vi "PQMain.vi"() -> ()   [LabVIEW 2009]
uses:
  PriorityQueue/Priority.ctl
  PriorityQueue/PriorityQueue.lvclass
  LinkedList/LinkedList.lvclass
panel:
  in  "Demo":enum32{"Basic", "Performance"}(tab)
  out "Message":string
  in  "Next Message":bool
  in  "Exit":bool
  out "data":i32(graph)
  out "generate (ms)":u32
  out "time enque":u32
  out "size":i32
  out "time deque":u32
  out "consume (ms)":u32
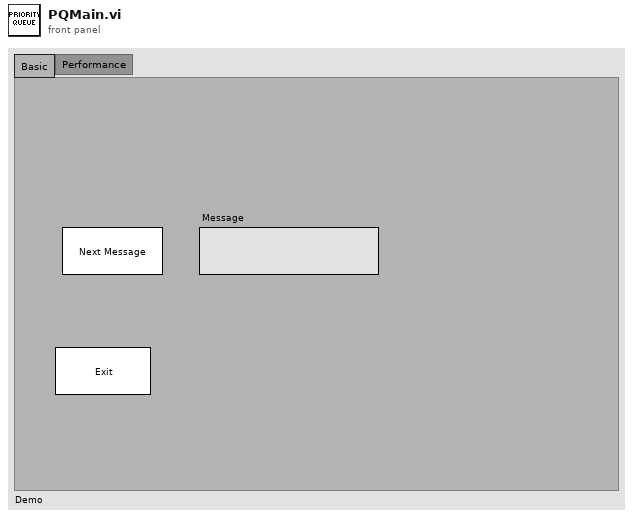
[diagram p1: front panel]
types:
  T1 = typedef "PriorityQueue.lvclass/Priority.ctl" = enum16{"High", "Medium", "Low"}
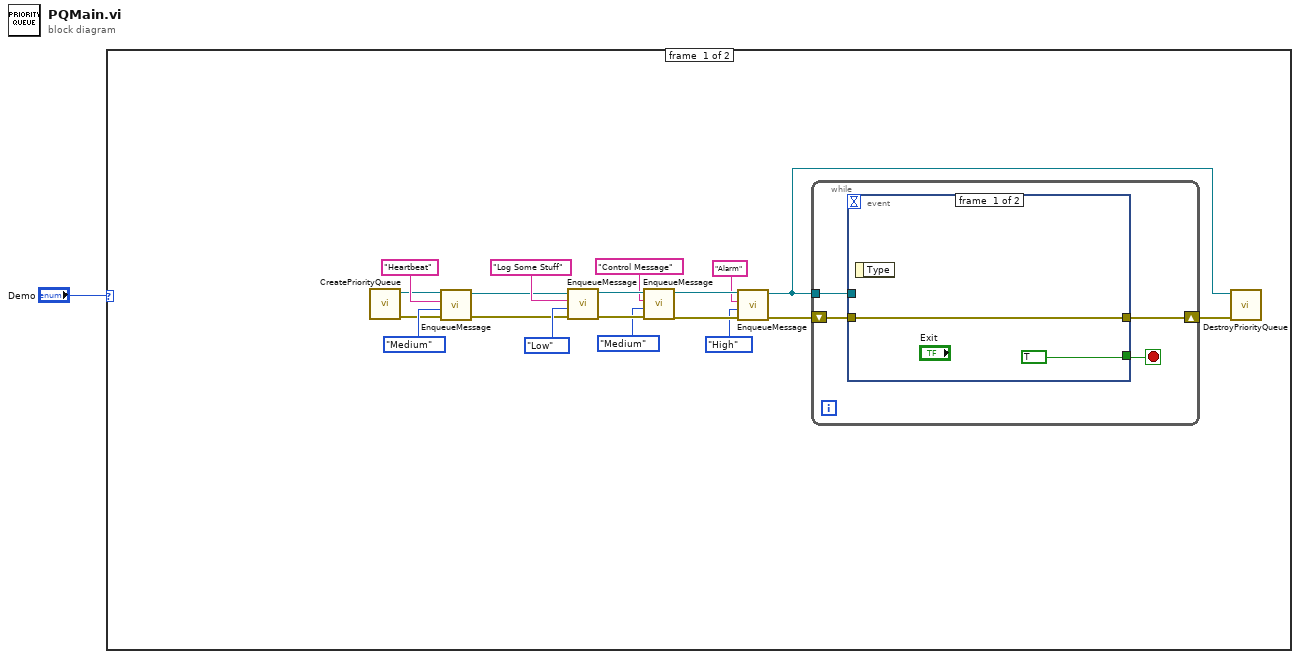
[diagram p0: block diagram]
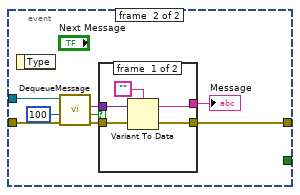
[diagram p2: hidden frame]
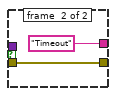
[diagram p3: hidden frame]
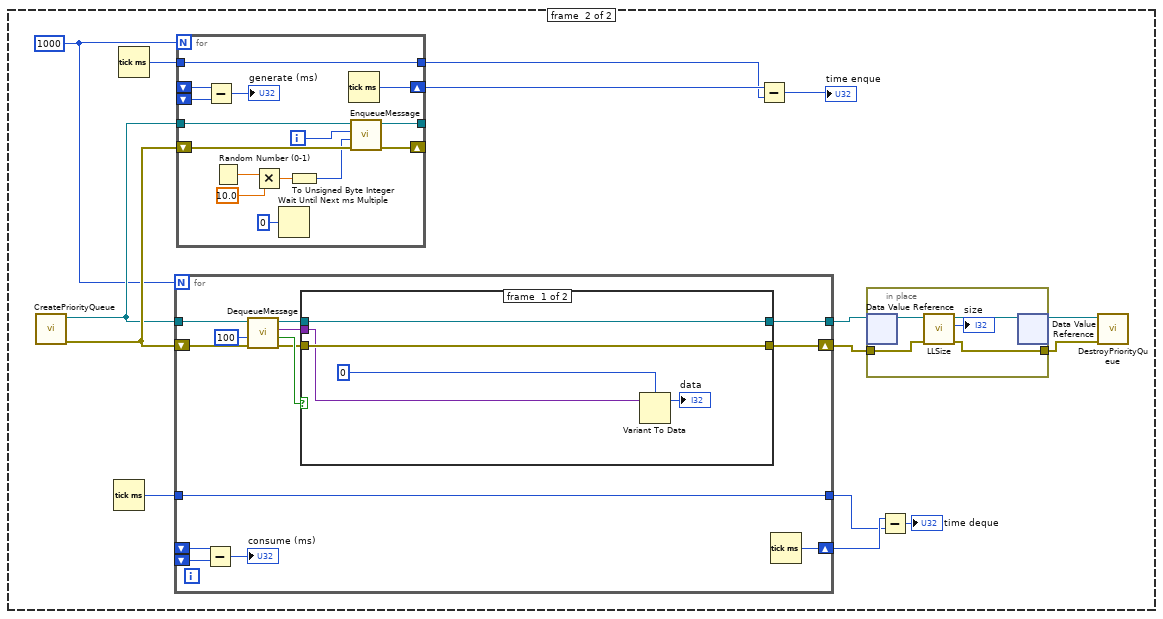
[diagram p4: hidden frame]
diagram:
  n1 = case shown="\"Basic\", Default" "Demo" {
    frame #0 {
      n2 = call "CreatePriorityQueue.vi"() -> ("error out"=w7:errorcluster, "PriorityQueue"=w6:refnum<data-value>)  [unwired: 10 in]
      n3 = call "EnqueueMessage.vi"("error in (no error)"=w7, "Priority"=Priority."Medium" ("Enum"), "message"="Heartbeat", "queue in"=w6) -> ("error out"=w4:errorcluster, "queue out"=w5:refnum<data-value>)  [unwired: 6 in]
      n4 = call "EnqueueMessage.vi"("error in (no error)"=w4, "Priority"=Priority."Low" ("Enum"), "message"="Log Some Stuff", "queue in"=w5) -> ("error out"=w19:errorcluster, "queue out"=w18:refnum<data-value>)  [unwired: 6 in]
      n5 = call "EnqueueMessage.vi"("error in (no error)"=w19, "Priority"=Priority."Medium" ("Enum"), "message"="Control Message", "queue in"=w18) -> ("error out"=w15:errorcluster, "queue out"=w16:refnum<data-value>)  [unwired: 6 in]
      n6 = call "EnqueueMessage.vi"("error in (no error)"=w15, "Priority"=Priority."High" ("Enum"), "message"="Alarm", "queue in"=w16) -> ("error out"=w3:errorcluster, "queue out"=w2:refnum<data-value>)  [unwired: 6 in]
      n7 = while {
        tunnel: w2 -> [w24]
        shift-right: [w22] -> w10
        shift-left: w3 -> [w23]
        stop <- w21 stop-if-true
        n8 = event shown="[1] \"Next Message\": Value Change" {
          selector: _ -> [_ _]
          dyn-events: _ -> [_ _]
          timeout: _ -> [_ _]
          tunnel: w24 -> [_ w34]
          tunnel: w23 -> [w26 w33]
          tunnel: [w26 w28] -> w22
          tunnel: [TRUE _] -> w21
          event #0 {
            n9 = event-data() -> ()  [unwired: 1 in, 1 out]
          }
          event #1 {
            n10 = event-data() -> ()  [unwired: 1 in, 1 out]
            n11 = call "DequeueMessage.vi"("error in (no error)"=w33, "ms timeout (-1)"=100, "queue in"=w34) -> ("error out"=w30:errorcluster, "timeout"=w31:bool, "message"=w29:variant)  [unwired: 5 in, 1 out]
            n12 = case shown="False" w31 {
              tunnel: w30 -> [w39 w41]
              tunnel: w29 -> [w37 _]
              tunnel: [w38 w41] -> w28
              tunnel: [w35 "Timeout" ("Message")] -> w27
              frame #0 {
                n13 = Variant To Data(error in=w39, Variant=w37, type="") -> (error out=w38:errorcluster, data=w35:string)
              }
              frame #1 {
              }
            }
            "Message" <- w27
          }
        }
      }
      n14 = call "DestroyPriorityQueue.vi"("error in (no error)"=w10, "Queue"=w2) -> ()  [unwired: 9 in, 1 out]
    }
    frame #1 {
      w49 = 1000
      n15 = call "CreatePriorityQueue.vi"() -> ("error out"=w51:errorcluster, "PriorityQueue"=w50:refnum<data-value>)  [unwired: 10 in]
      n16 = Tick Count (ms)() -> (millisecond timer value=w52:u32)
      n17 = Tick Count (ms)() -> (millisecond timer value=w56:u32)
      n18 = for {
        N: w49 -> [_]
        tunnel: w50 -> [w70]
        shift-right: [w63] -> w44
        shift-left: w51 -> [w69]
        tunnel: [w64] -> w45
        shift-right: [w62] -> w48
        shift-left: _ -> [w60]
        shift-left: _ -> [w61]
        tunnel: w52 -> [w58]
        tunnel: [w58] -> w47
        n19 = Subtract(x=w60, y=w61) -> (x-y=→"consume (ms)":u32)
        n20 = call "DequeueMessage.vi"("error in (no error)"=w69, "ms timeout (-1)"=100, "queue in"=w70) -> ("error out"=w66:errorcluster, "timeout"=w68:bool, "message"=w65:variant, "queue out"=w67:refnum<data-value>)  [unwired: 5 in]
        n21 = case shown="True" w68 {
          tunnel: w67 -> [w75 w77]
          tunnel: w66 -> [w74 w76]
          tunnel: w65 -> [w73 _]
          tunnel: [w75 w77] -> w64
          tunnel: [w74 w76] -> w63
          frame #0 {
            n22 = Variant To Data(Variant=w73, type=0) -> (data=→"data":i32)  [unwired: 1 in, 1 out]
          }
          frame #1 {
          }
        }
        n23 = Tick Count (ms)() -> (millisecond timer value=w62:u32)
      }
      n24 = for {
        N: w49 -> [_]
        tunnel: w50 -> [w97]
        shift-right: [w95] -> _
        shift-left: w51 -> [w96]
        shift-right: [w89] -> w55
        shift-left: _ -> [w87]
        shift-left: _ -> [w88]
        tunnel: [w85] -> _
        tunnel: w56 -> [w84]
        tunnel: [w84] -> w54
        i -> [w94]
        n25 = Subtract(x=w87, y=w88) -> (x-y=→"generate (ms)":u32)
        n26 = Random Number (0-1)() -> (number: 0 to 1=w93:dbl)
        n27 = Multiply(x=w93, y=10.0) -> (x*y=w91:dbl)
        n28 = Wait Until Next ms Multiple(millisecond multiple=u32 0) -> ()  [unwired: 1 out]
        n29 = To Unsigned Byte Integer(number=w91) -> (unsigned 8bit integer=w90:u8)
        n30 = Tick Count (ms)() -> (millisecond timer value=w89:u32)
        n31 = call "EnqueueMessage.vi"("error in (no error)"=w96, "Priority"=w90, "message"=w94, "queue in"=w97) -> ("error out"=w95:errorcluster, "queue out"=w85:refnum<data-value>)  [unwired: 6 in]
      }
      n32 = Subtract(x=w55, y=w54) -> (x-y=→"time enque":u32)
      n33 = in-place {
        in-place-border: w44 -> [w79]
        in-place-border: [w78] -> w43
        n34 = in-place-dvr #1(w45) -> (w82:refnum<class "PriorityQueue.lvclass">)  [unwired: 1 out]
        n35 = call "LLSize.vi"("error in (no error)"=w79, "LinkedList in"=w82) -> ("error out"=w78:errorcluster, "size"=→"size":i32, "LinkedList out"=w81:refnum<class "PriorityQueue.lvclass">)  [unwired: 7 in]
        n36 = in-place-dvr #1(w81) -> (w42:refnum<data-value>)  [unwired: 1 out]
      }
      n37 = Subtract(x=w48, y=w47) -> (x-y=→"time deque":u32)
      n38 = call "DestroyPriorityQueue.vi"("error in (no error)"=w43, "Queue"=w42) -> ()  [unwired: 9 in, 1 out]
    }
  }
